vi "Subscribing Groups.vi"(8 "error in (no error)":errorcluster, 11 "Group Data Handler in":refnum<class "Group Data Handler.lvclass">) -> (0 "error out":errorcluster, 2 "Subscribing Groups":string[](array[string]))   [LabVIEW 2020, in "VolatusHistorian.lvlib" / "Group Data Handler.lvclass"]
uses:
  Group Data Handler.lvclass
  Group Data Handler.lvclass/Group Data Handler.ctl
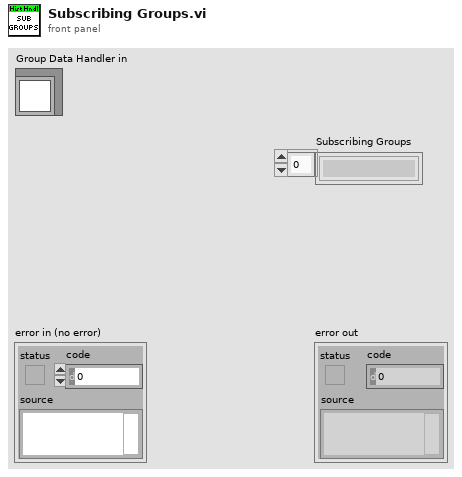
[diagram p1: front panel]
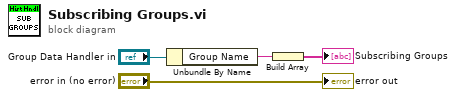
[diagram p0: block diagram]
diagram:
  n1 = Unbundle By Name("Group Data Handler in") -> ("Group Name"=w2:string)
  n2 = Build Array(w2) -> (→"Subscribing Groups":string[])
  "error out" <- "error in (no error)"
